vi "ListeMatCSRToArray.vi"(8 "error in":errorcluster caption="entrée d'erreur", 11 "Liste de la matrice creuse":string) -> (0 "error out":errorcluster caption="sortie d'erreur", 3 "StringSparse 2DArray":string[][](array[string]))   [LabVIEW 2020]
uses:
  <vilib>/Utility/error.llb/Error Cluster From Error Code.vi
  <vilib>/ErrorRing/Error Ring.xnode
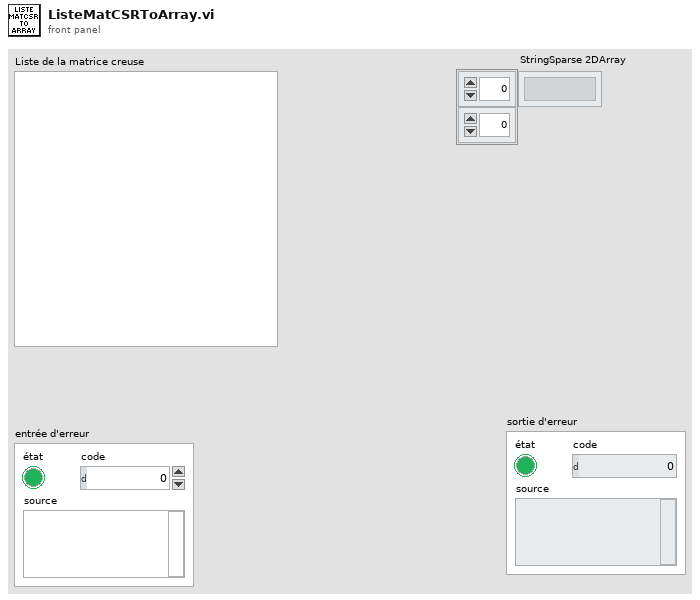
[diagram p1: front panel]
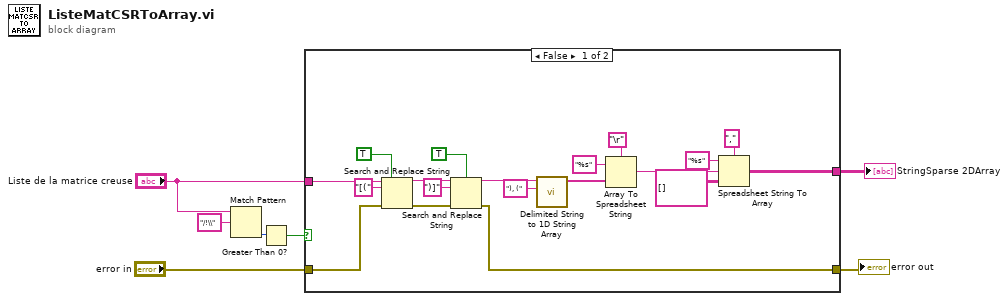
[diagram p0: block diagram]
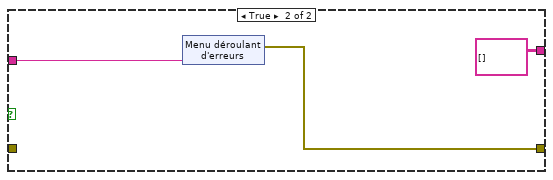
[diagram p2: hidden frame]
diagram:
  n1 = Match Pattern(string="Liste de la matrice creuse", regular expression="/!\\" ("expression régulière")) -> (offset past match=w6:i32)  [unwired: 1 in, 3 out]
  n2 = Greater Than 0?(x=w6) -> (x > 0?=w4:bool)
  n3 = case shown="False" w4 {
    tunnel: "Liste de la matrice creuse" -> [w26 w28]
    tunnel: [w11 string[][] []] -> w3
    tunnel: "error in" -> [w10 _]
    tunnel: [w8 w27] -> w1
    frame False {
      n4 = Search and Replace String(replace all?=TRUE ("tout remplacer ? (F)"), input string=w26, search string="[(" ("chaîne recherchée"), error in=w10) -> (result string=w23:string, error out=w9:errorcluster)  [unwired: 4 in, 2 out]
      n5 = Search and Replace String(case sensitive?=TRUE ("ignorer la casse ? (F)"), input string=w23, search string=")]" ("chaîne recherchée"), error in=w9) -> (result string=w20:string, error out=w8:errorcluster)  [unwired: 4 in, 2 out]
      n6 = call <vilib>:"Delimited String to 1D String Array.vi"("delimiter"="), (", "delimited string"=w20) -> ("string array"=w13:string[])  [unwired: 9 in]
      n7 = Array To Spreadsheet String(delimiter (Tab)="\r", array=w13, 3:"%s" ("chaîne de format")) -> (spreadsheet string=w12:string)
      n8 = Spreadsheet String To Array(delimiter (Tab)="," ("séparateur (Tabulation)"), format string="%s" ("chaîne de format"), spreadsheet string=w12, array type (2D Dbl)=string[][] []) -> (array=w11:string[][])
    }
    frame True {
      n9 = xnode "Menu déroulant d'erreurs"("parameter 0"=w28) -> ("error out"=w27:errorcluster)
    }
  }
  "StringSparse 2DArray" <- w3
  "error out" <- w1
